vi "Copy Instrumentstudio Template.vi"(8 "error in (no error)":errorcluster) -> (0 "error out":errorcluster)   [LabVIEW 2021, in "Converter.lvlib"]
uses:
  Converter.lvlib
  Path Functions/Path Functions.lvlib
  <vilib>/ErrorRing/Error Ring.xnode
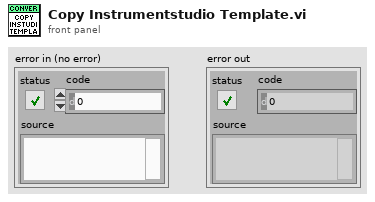
[diagram p1: front panel]
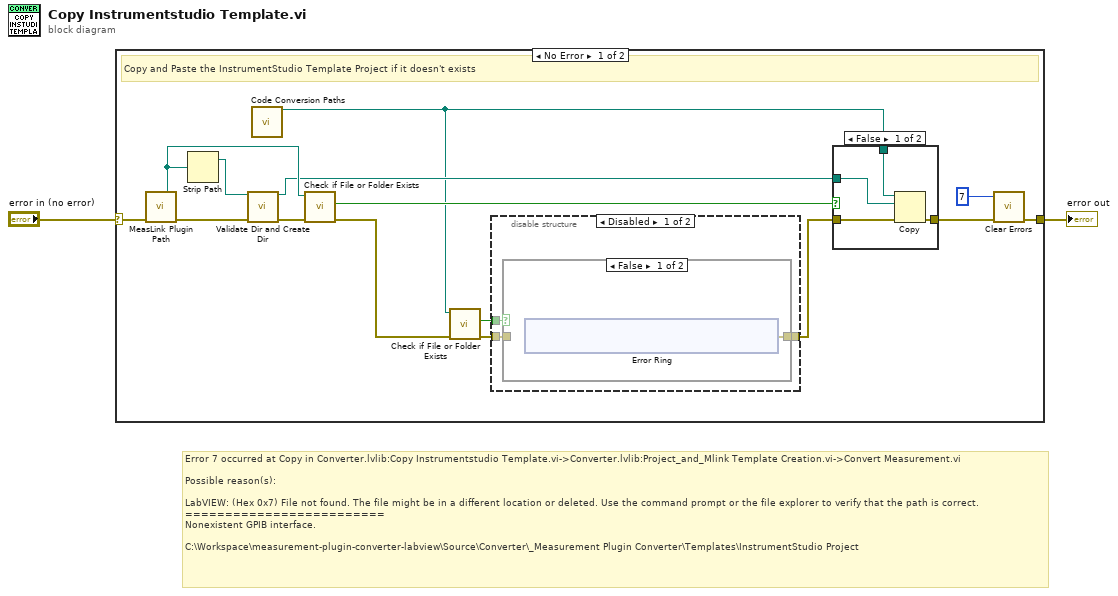
[diagram p0: block diagram]
diagram:
  # "Error 7 occurred at Copy in Converter.lvlib:Copy Instrumentstudio Template.vi->Converter.lvlib:Project_and_Mlink Template Creation.vi->Convert Measurement.vi\n\nPossible reason(s):\n\nLabVIEW: (Hex 0x7) File not found. The file might be in a different location or deleted. Use the command prompt or the file explorer to verify that the path is correct.\n=========================\nNonexistent GPIB interface.\n\nC:\\Workspace\\measurement-plugin-converter-labview\\Source\\Converter\\_Measurement Plugin Converter\\Templates\\InstrumentStudio Project"
  n1 = case shown="No Error" "error in (no error)" {
    selector: "error in (no error)" -> [w17 w30]
    tunnel: [w4 w30] -> w1
    frame No Error {
      # "Copy and Paste the InstrumentStudio Template Project if it doesn't exists"
      n2 = call "MeasLink Plugin Path.vi"("error in (no error)"=w17) -> ("Instrumentstudio Folder"=w15:path, "error out"=w11:errorcluster)  [unwired: 2 in, 11 out]
      n3 = Strip Path(path=w15) -> (stripped path=w13:path)  [unwired: 1 out]
      n4 = call "Validate Dir and Create Dir.vi"("Directory"=w13, "error in (no error)"=w11) -> ("Dup Directory"=w12:path, "error out"=w10:errorcluster)  [unwired: 12 in]
      n5 = call "Code Conversion Paths.vi"() -> ("IS Project Directory"=w5:path)  [unwired: 7 in, 8 out]
      n6 = call <vilib>:"Check if File or Folder Exists.vi"("error in (no error)"=w10, "path"=w15) -> ("error out"=w7:errorcluster, "file or folder exists?"=w14:bool)  [unwired: 7 in, 1 out]
      n7 = call <vilib>:"Check if File or Folder Exists.vi"("error in (no error)"=w7, "path"=w5) -> ("error out"=w9:errorcluster, "file or folder exists?"=w8:bool)  [unwired: 7 in, 1 out]
      n8 = disable-structure shown="Disabled" {
        disable-tunnel: w9 -> [w20 w24]
        disable-tunnel: w8 -> [w19 _]
        disable-tunnel: [w18 w24] -> w6
        frame Disabled {
          n9 = case shown="False" w19 {
            tunnel: w20 -> [_ w23]
            tunnel: [w21 w23] -> w18
            frame False {
              n10 = xnode "Error Ring"() -> ("error out"=w21:errorcluster)
            }
            frame True {
            }
          }
        }
        frame Enabled {
        }
      }
      n11 = case shown="False" w14 {
        tunnel: [w28 w29] -> w16
        tunnel: w5 -> [w27 _]
        tunnel: w12 -> [w26 _]
        tunnel: w6 -> [w25 w29]
        frame False {
          n12 = Copy(8:w25, 10:w26, 11:w27) -> (0:w28:errorcluster)  [unwired: 4 out]
        }
        frame True {
        }
      }
      n13 = call <vilib>:"Clear Errors.vi"("error in (no error)"=w16, "specific error code to clear (0: all)"=7) -> ("error out"=w4:errorcluster)  [unwired: 4 in, 1 out]
    }
    frame Error {
    }
  }
  "error out" <- w1
